vi "Pfeiffer-RVC300.open valve.vi"(0 "i ref in":refnum<vi>, 3 "ms timeout (10000)":i32=10000, 5 "error in (no error)":errorcluster) -> (14 "i ref out":refnum<vi>, 17 "timed out":bool, 19 "error out":errorcluster)   [LabVIEW 2014, in "Pfeiffer-RVC300.lvlib"]
doc: "Opens the valve completely (be careful!).\n\nLicense Agreement for this software:\n\nCopyright (C)\nMax-Planck-Institut für Kernphysik\nSaupfercheckweg 1\n69117 Heidelberg\nGermany\n\nContact: christopher.borgmann@mpi-hd.mpg.de\n\nThis program is free software: you can redistribute it and/or modify \nit under the terms of the GNU General Public License as published by\nthe Free Software Foundation, either version 3 of the License, or\n(at your option) any later version.\n\nThis program is distributed in the hope that it will be useful,\nbut WITHOUT ANY WARRANTY; without even the implied warranty of\nMERCHANTABILITY or FITNESS FOR A PARTICULAR PURPOSE. See the\nGNU General Public License for more details.\n\nYou should have received a copy of the GNU General Public License\nalong with this program. If not, see <http://www.gnu.org/licenses/>.\n\nMax-Planck-Institut für Kernphysik\nSaupfercheckweg 1, 69117 Heidelberg, Germany\nFor all questions and ideas contact: christopher.borgmann@mpi-hd.mpg.de\nLast update: 08.07.2010"
uses:
  Pfeiffer-RVC300.lvlib
  CS_Core/CSApplicationBaseClasses/DeviceBase/DeviceBase.lvlib
  instr.lib/RVC300/RVC 300.lvlib
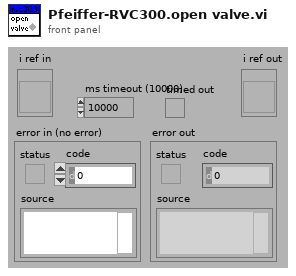
[diagram p1: front panel]
types:
  T1 = typedef "Pfeiffer-RVC300.lvlib/Pfeiffer-RVC300.i attribute.ctl" = cluster{"interfaceInitialized":bool, "VISAResource":refnum<visa-resource-name>, "WaitingTime":u32, "nomValues":T2, "actValues":T2}
  T2 = typedef "Pfeiffer-RVC300.lvlib/Pfeiffer-RVC300.parameters.ctl" = cluster{"regulationMode":T3, "valveType":string, "sensorType":string, "valveState":string, "flow":dbl, "pressure":dbl, "serviceIDs":cluster{"regulationModeID":i32, "valveTypeID":i32, "sensorTypeID":i32, "valveStateID":i32, "flowID":i32, "pressureID":i32}}
  T3 = typedef "Pfeiffer-RVC300.lvlib/Pfeiffer-RVC300.regulation mode.ctl" = enum16{"unknown", "Pressure", "Flow", "Wait"}
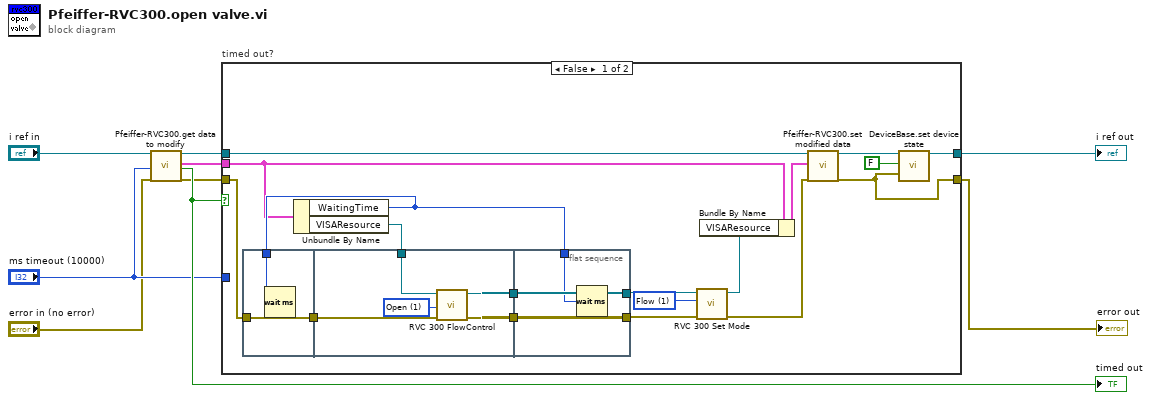
[diagram p0: block diagram]
diagram:
  n1 = call "Pfeiffer-RVC300.get data to modify.vi"("i ref in"="i ref in", "ms timeout (10000)"="ms timeout (10000)", "error in (no error)"="error in (no error)") -> ("i ref out"=w3:refnum<vi>, "i attribute"=w1:T1, "timed out"=w6:bool, "error out"=w2:errorcluster)  [unwired: 13 in]
  "timed out" <- w6
  n2 = case "timed out?" shown="False" w6 {
    tunnel: [w25 w39] -> w8
    tunnel: w3 -> [w27 w39]
    tunnel: [w23 w38] -> w7
    tunnel: w2 -> [w13 w38]
    tunnel: w1 -> [w11 _]
    tunnel: "ms timeout (10000)" -> [_ _]
    frame False {
      w16 = u16 1 items=["Pressure", "Flow", "Wait"] ("Mode")
      n3 = flat-sequence {
        tunnel: w13 -> [w29]
        tunnel: [w29] -> w22
        tunnel: w14 -> [w28]
        tunnel: [w33] -> w21
        tunnel: [w31] -> w20
        tunnel: w22 -> [w34]
        tunnel: w15 -> [w30]
        tunnel: [w36] -> w18
        tunnel: [w37] -> w19
        tunnel: w21 -> [w37]
        tunnel: w20 -> [w36]
        tunnel: w14 -> [w35]
        frame #0 {
          n4 = Wait (ms)(milliseconds to wait=w28) -> ()  [unwired: 1 out]
        }
        frame #1 {
          w32 = u16 1 items=["Close", "Open", "Control"] ("Action")
          n5 = call "RVC 300 FlowControl.vi"("error in"=w34, "Action"=w32, "Resource Name"=w30) -> ("error out"=w31:errorcluster, "Resource Name out"=w33:refnum<visa-resource-name>)  [unwired: 6 in, 1 out]
        }
        frame #2 {
          n6 = Wait (ms)(milliseconds to wait=w35) -> ()  [unwired: 1 out]
        }
      }
      n7 = Unbundle By Name(w11) -> ("WaitingTime"=w14:u32, "VISAResource"=w15:refnum<visa-resource-name>)
      n8 = call "RVC 300 Set Mode.vi"("error in"=w18, "Mode"=w16, "Resource Name"=w19) -> ("error out"=w12:errorcluster, "Resource Name out"=w17:refnum<visa-resource-name>)  [unwired: 3 in]
      n9 = Bundle By Name(cluster=w11, "VISAResource"=w17) -> (w10:T1)
      n10 = call "Pfeiffer-RVC300.set modified data.vi"("i ref in"=w27, "i attribute"=w10, "error in (no error)"=w12) -> ("i ref out"=w26:refnum<vi>, "error out"=w23:errorcluster)  [unwired: 15 in]
      n11 = call "DeviceBase.set device state.vi"("i ref in"=w26, "implicit"=FALSE, "device error"=w23) -> ("i ref out"=w25:refnum<vi>)  [unwired: 14 in, 2 out]
    }
    frame True {
    }
  }
  "error out" <- w7
  "i ref out" <- w8
